vi "LNLS Control Encode LOCON_BIPOLAR_16BITS.vi"(8 "error in (no error)":errorcluster, 11 "LOCON Data":T1[](array[typedef]) {"status" format="%08b"}) -> (0 "error out":errorcluster, 2 "command body":string)   [LabVIEW 2011, in "LNLS Control VIs.lvlib"]
uses:
  LNLS Control VIs.lvlib
  Types Definitions/Type LOCON_BIPOLAR_16BITS.ctl
  Type Definitions.lvlib
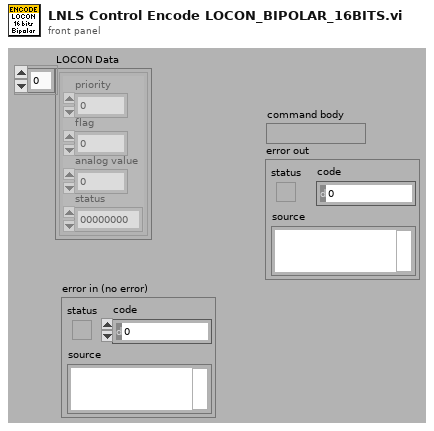
[diagram p1: front panel]
types:
  T1 = typedef "Type Definitions.lvlib/Type LOCON_BIPOLAR_16BITS.ctl" = cluster{"priority":u8, "flag":u8, "analog value":u16, "status":u8}
  T2 = enum16{"big-endian, network order", "native, host order", "little-endian"}
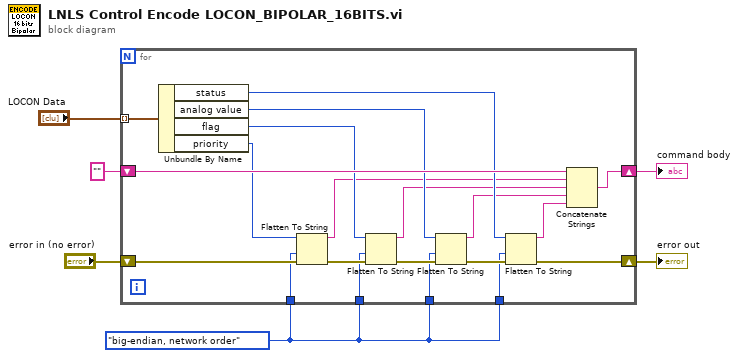
[diagram p0: block diagram]
diagram:
  w2 = T2."big-endian, network order" ("byte order (0:big-endian, network order)")
  n1 = for {
    shift-right: [w22] -> w5
    shift-left: "error in (no error)" -> [w21]
    tunnel: "LOCON Data" -> [w26] mode=indexing
    shift-right: [w20] -> w4
    shift-left: "" -> [w19]
    tunnel: w2 -> [w10]
    tunnel: w2 -> [w9]
    tunnel: w2 -> [w8]
    tunnel: w2 -> [w7]
    n2 = Unbundle By Name(w26) -> ("status"=w15:u8, "analog value"=w16:u16, "flag"=w17:u8, "priority"=w18:u8)
    n3 = Flatten To String(anything=w18, byte order (0:big-endian, network order)=w7, error in (no error)=w21) -> (data string=w14:string, error out=w25:errorcluster)  [unwired: 1 in, 1 out]
    n4 = Flatten To String(anything=w17, byte order (0:big-endian, network order)=w8, error in (no error)=w25) -> (data string=w13:string, error out=w24:errorcluster)  [unwired: 1 in, 1 out]
    n5 = Flatten To String(anything=w16, byte order (0:big-endian, network order)=w9, error in (no error)=w24) -> (data string=w12:string, error out=w23:errorcluster)  [unwired: 1 in, 1 out]
    n6 = Flatten To String(anything=w15, byte order (0:big-endian, network order)=w10, error in (no error)=w23) -> (data string=w11:string, error out=w22:errorcluster)  [unwired: 1 in, 1 out]
    n7 = Concatenate Strings(w19, w14, w13, w12, w11) -> (w20:string)
  }
  "command body" <- w4
  "error out" <- w5
